vi "ConvertTextBoxToNumericalArray.vi"(8 "Error In":errorcluster, 11 "Configuration Commands":string="Register,Register Value\r4603,2\r4604,10") -> (0 "Error Out":errorcluster, 2 "Register Value":u16[](array[numeric]), 3 "Register":u16[](array[numeric]))   [LabVIEW 2018, in "SensorPlugins.lvlib" / "SiemensDigitalEnergyMeter.lvclass"]
uses:
  SiemensDigitalEnergyMeter.lvclass
panel:
  out "SpreadsheetArray":string[][](array[string])
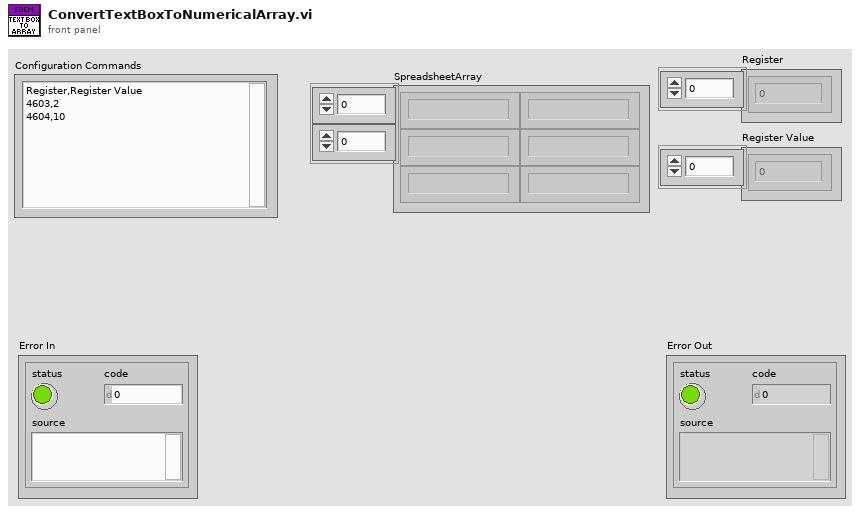
[diagram p1: front panel]
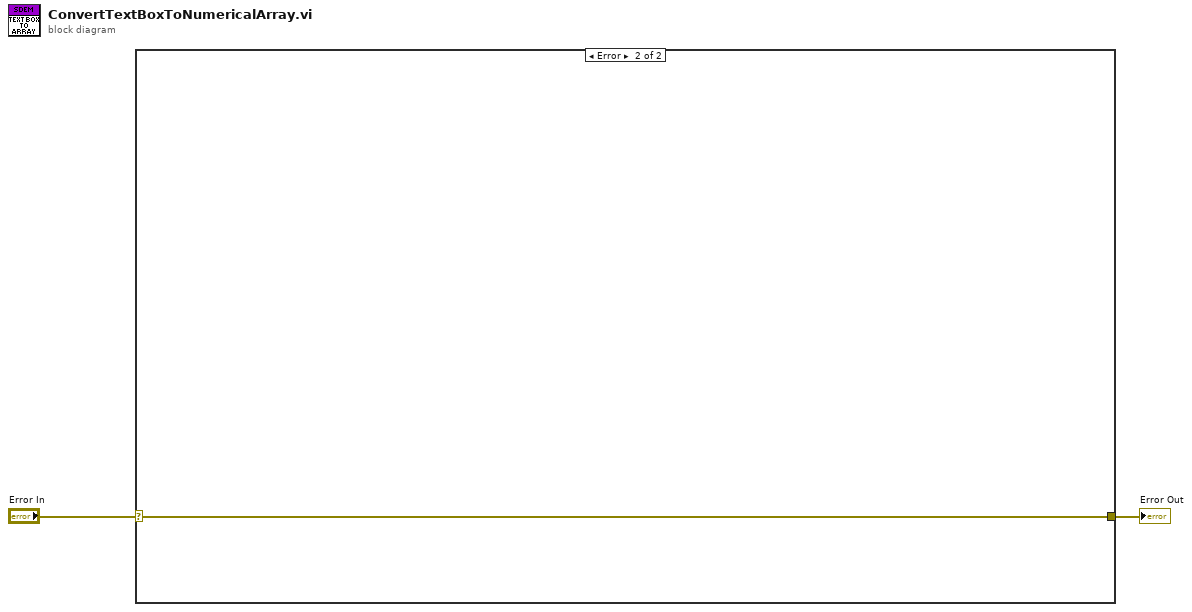
[diagram p0: block diagram]
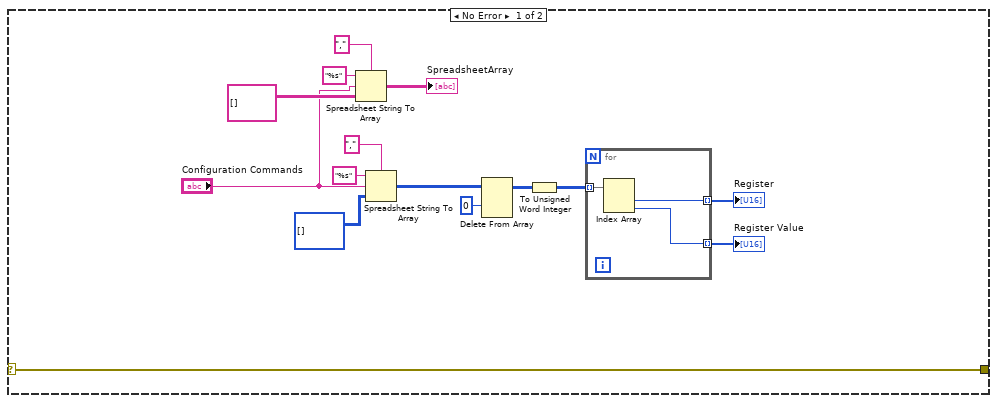
[diagram p2: hidden frame]
diagram:
  n1 = case shown="Error" "Error In" {
    selector: "Error In" -> [w3 w21]
    tunnel: [w3 w21] -> w1
    frame No Error {
      n2 = Spreadsheet String To Array(delimiter (Tab)=",", format string="%s", spreadsheet string="Configuration Commands", array type (2D Dbl)=string[][] [] ("unsigned 16bit integer")) -> (array=→"SpreadsheetArray":string[][])
      n3 = Spreadsheet String To Array(delimiter (Tab)=",", format string="%s", spreadsheet string="Configuration Commands", array type (2D Dbl)=u16[][] [] ("unsigned 16bit integer")) -> (array=w11:u16[][])
      n4 = Delete From Array(array=w11, index (row)=0) -> (array with subset deleted=w13:u16[][])  [unwired: 2 in, 1 out]
      n5 = To Unsigned Word Integer(number=w13) -> (unsigned 16bit integer=w10:u16[][])
      n6 = for {
        tunnel: w10 -> [w20] mode=indexing
        tunnel: [w19] -> w15 mode=indexing
        tunnel: [w18] -> w14 mode=indexing
        n7 = Index Array(array=w20) -> (element #1=w19:u16, element #2=w18:u16)  [unwired: 2 in]
      }
      "Register" <- w15
      "Register Value" <- w14
    }
    frame Error {
    }
  }
  "Error Out" <- w1
